vi "OxITC503 _Config_ Read or Write AUTO-PIDTable.vi"(3 "error in":errorcluster, 4 "AUTO-PID Table in":T2(array[cluster]) {"Derivative Action Time" format="%.1f"; "Integral Action Time" format="%.1f"; "Proportional Band" format="%.3f"; "Upper Bound Temperature" format="%.3f"}, 5 "Operation (read)":T1(ring), 6 "VISA session in":refnum<visa-resource-name>) -> (0 "error out":errorcluster, 1 "AUTO-PID Table out":T2(array[cluster]) {"Derivative Action Time" format="%.1f"; "Integral Action Time" format="%.1f"; "Proportional Band" format="%.3f"; "Upper Bound Temperature" format="%.3f"}, 2 "VISA session out":refnum<visa-resource-name>)   [LabVIEW 2013]
doc: "Reads/writes AUTO-PID table."
panel:
  out "Message":string
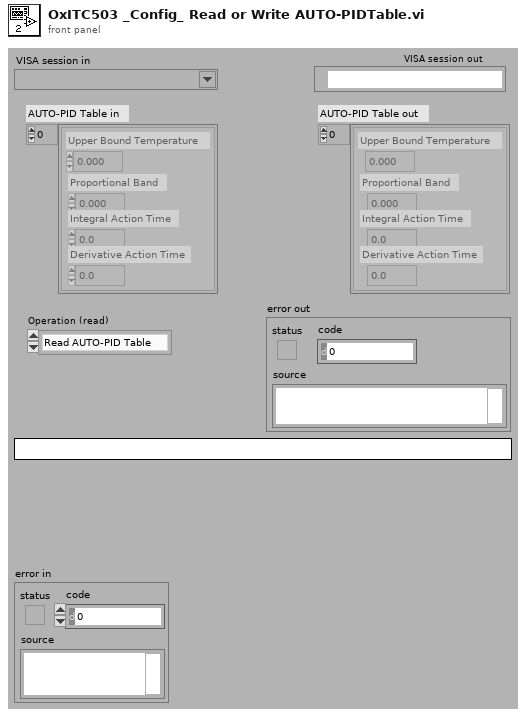
[diagram p1: front panel]
types:
  T1 = enum16{"Read AUTO-PID Table", "Write AUTO-PID Table"}
  T2 = cluster{"Upper Bound Temperature":dbl, "Proportional Band":dbl, "Integral Action Time":dbl, "Derivative Action Time":dbl}[]
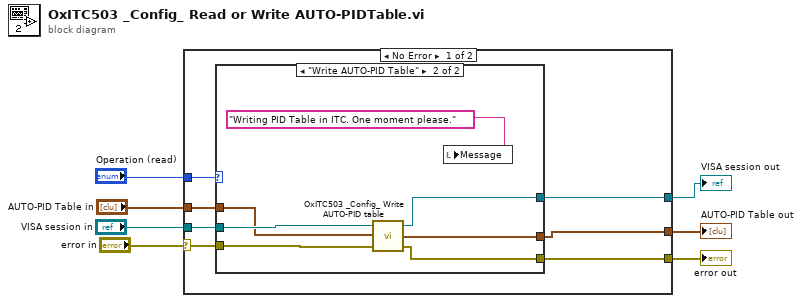
[diagram p0: block diagram]
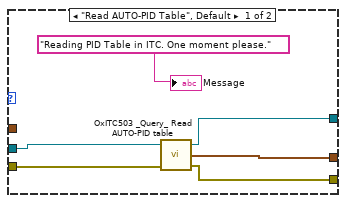
[diagram p2: hidden frame]
diagram:
  n1 = case shown="No Error" "error in" {
    selector: "error in" -> [w12 w29]
    tunnel: "VISA session in" -> [w14 w30]
    tunnel: "Operation (read)" -> [w13 _]
    tunnel: [w11 w30] -> w5
    tunnel: [w10 w29] -> w4
    tunnel: "AUTO-PID Table in" -> [w9 w28]
    tunnel: [w8 w28] -> w2
    frame No Error {
      n2 = case shown="\"Write AUTO-PID Table\"" w13 {
        tunnel: w14 -> [w19 w26]
        tunnel: w12 -> [w18 w25]
        tunnel: [w17 w24] -> w8
        tunnel: [w16 w23] -> w11
        tunnel: [w15 w22] -> w10
        tunnel: w9 -> [_ w21]
        frame "Read AUTO-PID Table", Default {
          n3 = call "OxITC503 _Query_ Read AUTO-PID table.vi"("error in"=w18, "VISA session in"=w19) -> ("error out"=w15:errorcluster, "AUTOPID Table out"=w17:T2, "VISA session ou"=w16:refnum<visa-resource-name>)  [unwired: 1 in]
          "Message" <- "Reading PID Table in ITC. One moment please."
        }
        frame "Write AUTO-PID Table" {
          n4 = call "OxITC503 _Config_ Write AUTO-PID table.vi"("error in"=w25, "AUTOPID Table in"=w21, "VISA session in"=w26) -> ("error out"=w22:errorcluster, "AUTOPID Table out"=w24:T2, "VISA session out"=w23:refnum<visa-resource-name>)
          n5 = local write "Message"("Writing PID Table in ITC. One moment please.") -> ()
        }
      }
    }
    frame Error {
    }
  }
  "VISA session out" <- w5
  "error out" <- w4
  "AUTO-PID Table out" <- w2
